vi "SSS_TX_GENERATE (SubVI).vi"(4 "초기 위상":dbl format="%#_13g", 6 "Start Frequency(Hz)":dbl=430000.0 format="%#_6p", 7 "Bandwidth":dbl=40000.0 format="%#_6p", 9 "sampling rate":dbl=3760000.0 caption="Sampling Frequency" format="%0.2f", 10 "Pulse length(sec)":dbl=4e-06, 11 "STEP":i32=100) -> (1 "TX.CH1 2":waveform(dbl)(graph), 2 "TX Spectrum":cluster{"f0":dbl, "df":dbl, "magnitude":dbl[]}(graph), 3 "TX.CH1":waveform(dbl)(graph), 5 "Hz/1STEP":dbl)   [LabVIEW 2017]
uses:
  <vilib>/measure/maspectr.llb/FFT Power Spectrum and PSD for 1 Chan.vi
  <vilib>/Analysis/NI_AALBase.lvlib
  <vilib>/measure/NI_MAPro.lvlib
panel:
  out "크기 2":i32
  out "크기":i32
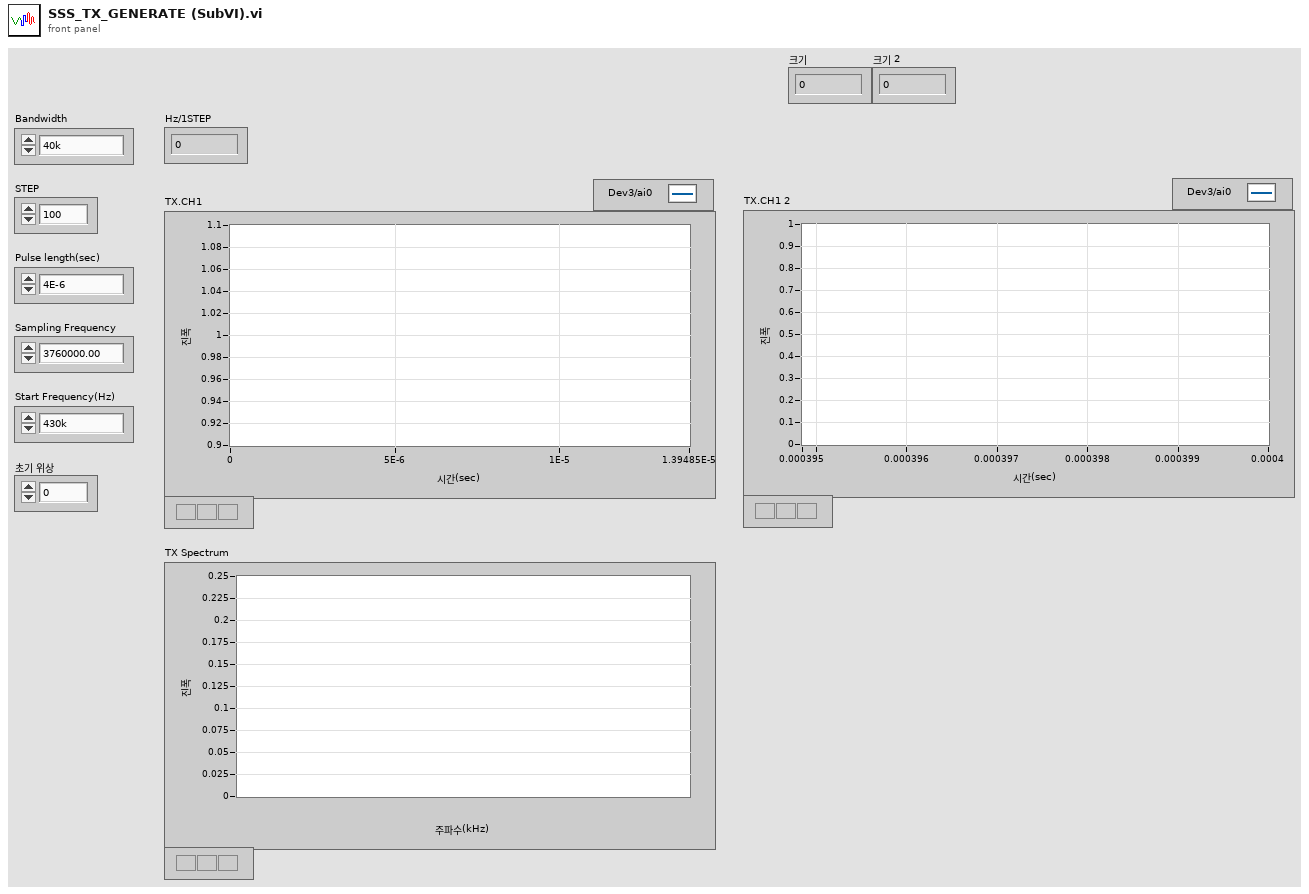
[diagram p1: front panel]
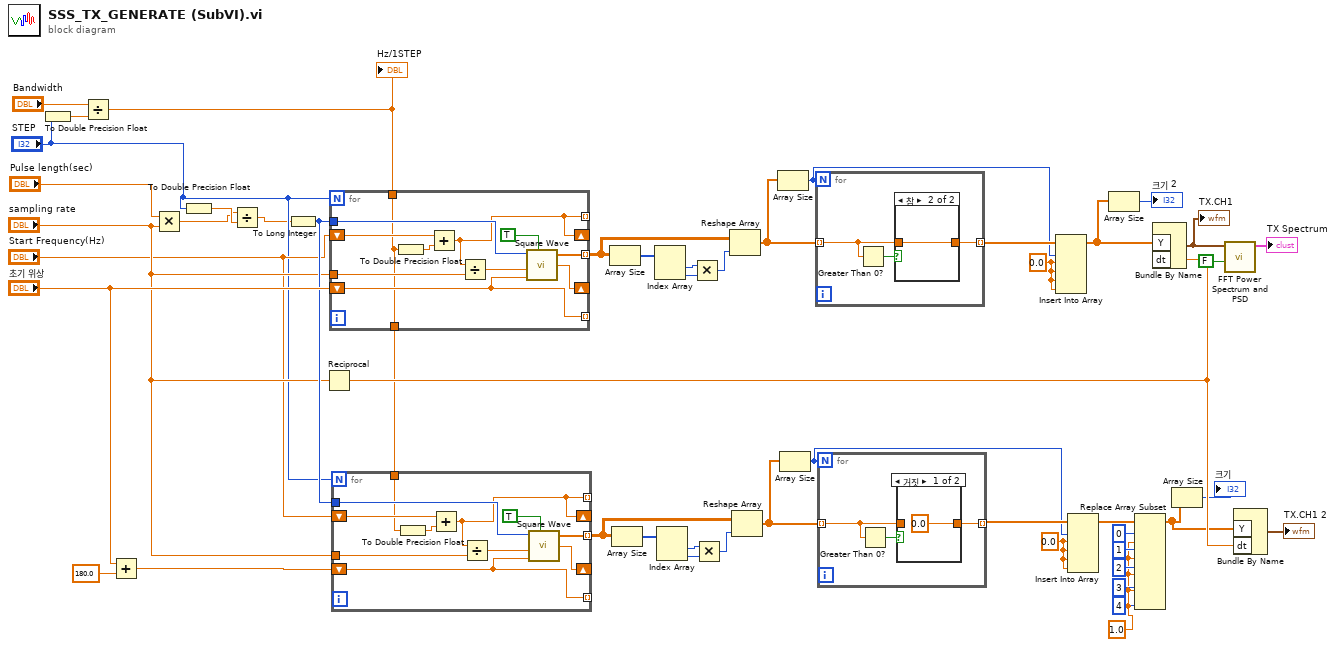
[diagram p0: block diagram]
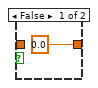
[diagram p3: hidden frame]
diagram:
  w9 = 1.0 ("새 원소/부분배열")
  w18 = 0.0 ("새 원소/부분배열")
  w19 = 0.0 ("새 원소/부분배열")
  n1 = To Double Precision Float(number="STEP") -> (double precision float=w33:dbl)
  n2 = Divide(x="Bandwidth", y=w33) -> (x/y=w34:dbl)
  "Hz/1STEP" <- w34
  n3 = Add(x="초기 위상", y=180.0) -> (x+y=w47:dbl)
  n4 = Multiply(x="Pulse length(sec)", y="sampling rate") -> (x*y=w2:dbl)
  n5 = To Double Precision Float(number="STEP") -> (double precision float=w3:dbl)
  n6 = Divide(x=w2, y=w3) -> (x/y=w1:dbl)
  n7 = To Long Integer(number=w1) -> (32bit integer=w43:i32)
  n8 = Reciprocal(x="sampling rate") -> (1/x=w48:dbl)
  n9 = for {
    N: "STEP" -> [_]
    tunnel: w43 -> [w60]
    shift-right: [w58] -> _
    shift-left: "초기 위상" -> [w51]
    tunnel: [w57] -> w25 mode=indexing
    shift-right: [w52] -> _
    shift-left: "Start Frequency(Hz)" -> [w56]
    tunnel: "sampling rate" -> [w54]
    tunnel: [w52] -> _ mode=indexing
    tunnel: [w51] -> _ mode=indexing
    tunnel: w34 -> [w50]
    tunnel: [w50] -> w44
    n10 = To Double Precision Float(number=w50) -> (double precision float=w55:dbl)
    n11 = Add(x=w56, y=w55) -> (x+y=w52:dbl)
    n12 = Divide(x=w52, y=w54) -> (x/y=w53:dbl)
    n13 = call <vilib>:"Square Wave.vi"("samples"=w60, "reset phase"=TRUE, "frequency"=w53, "phase in"=w51) -> ("square wave"=w57:dbl[], "phase out"=w58:dbl)  [unwired: 2 in, 1 out]
  }
  n14 = for {
    N: "STEP" -> [_]
    tunnel: w43 -> [w71]
    shift-right: [w69] -> _
    shift-left: w47 -> [w62]
    tunnel: [w68] -> w37 mode=indexing
    shift-right: [w63] -> _
    shift-left: "Start Frequency(Hz)" -> [w67]
    tunnel: "sampling rate" -> [w65]
    tunnel: [w63] -> _ mode=indexing
    tunnel: [w62] -> _ mode=indexing
    tunnel: w44 -> [w61]
    n15 = To Double Precision Float(number=w61) -> (double precision float=w66:dbl)
    n16 = Add(x=w67, y=w66) -> (x+y=w63:dbl)
    n17 = Divide(x=w63, y=w65) -> (x/y=w64:dbl)
    n18 = call <vilib>:"Square Wave.vi"("samples"=w71, "reset phase"=TRUE, "frequency"=w64, "phase in"=w62) -> ("square wave"=w68:dbl[], "phase out"=w69:dbl)  [unwired: 2 in, 1 out]
  }
  n19 = Array Size(array=w25) -> (size(s)=w24:i32[])
  n20 = Array Size(array=w37) -> (size(s)=w36:i32[])
  n21 = Index Array(array=w24) -> (element #1=w26:i32, element #2=w27:i32)  [unwired: 2 in]
  n22 = Index Array(array=w36) -> (element #1=w38:i32, element #2=w39:i32)  [unwired: 2 in]
  n23 = Multiply(x=w26, y=w27) -> (x*y=w23:i32)
  n24 = Multiply(x=w38, y=w39) -> (x*y=w35:i32)
  n25 = Reshape Array(w25, w23) -> (w31:dbl[])
  n26 = Reshape Array(w37, w35) -> (w40:dbl[])
  n27 = Array Size(array=w31) -> (size(s)=w20:i32)
  n28 = Array Size(array=w40) -> (size(s)=w16:i32)
  n29 = for {
    N: w20 -> [_]
    tunnel: w31 -> [w73] mode=indexing
    tunnel: [w72] -> w21 mode=indexing
    n30 = Greater Than 0?(x=w73) -> (x > 0?=w74:bool)
    n31 = case shown="참" w74 {
      tunnel: w73 -> [_ w76]
      tunnel: [0.0 w76] -> w72
      frame False {
      }
      frame True {
      }
    }
  }
  n32 = for {
    N: w16 -> [_]
    tunnel: w40 -> [w78] mode=indexing
    tunnel: [w77] -> w17 mode=indexing
    n33 = Greater Than 0?(x=w78) -> (x > 0?=w79:bool)
    n34 = case shown="거짓" w79 {
      tunnel: w78 -> [_ w81]
      tunnel: [0.0 w81] -> w77
      frame False {
      }
      frame True {
      }
    }
  }
  n35 = Insert Into Array(array=w21, index=w20, new element #1=w19, new element #2=w19, new element #3=w19, new element #4=w19) -> (w6:dbl[])
  n36 = Insert Into Array(array=w17, index=w16, new element #1=w18, new element #2=w18, new element #3=w18, new element #4=w18) -> (w15:dbl[])
  n37 = Array Size(array=w6) -> (size(s)=→"크기 2":i32)
  n38 = Replace Array Subset(array=w15, new element #1=w9, index #1=0 ("인덱스"), new element #2=w9, index #2=1 ("인덱스"), new element #3=w9, index #3=2 ("인덱스"), new element #4=w9, index #4=3 ("인덱스"), new element #5=w9, index #5=4 ("인덱스")) -> (w8:dbl[])
  n39 = Bundle By Name("Y"=w6, "dt"=w48) -> (w29:waveform(dbl))  [unwired: 1 in]
  "TX.CH1" <- w29
  n40 = Array Size(array=w8) -> (size(s)=→"크기":i32)
  n41 = call-poly <vilib>:"FFT Power Spectrum and PSD.vi"("dB On (F)"=FALSE, "time signal"=w29) -> ("Power Spectrum / PSD"=→"TX Spectrum":cluster{"f0":dbl, "df":dbl, "magnitude":dbl[]})  [unwired: 6 in, 3 out]
  n42 = Bundle By Name("Y"=w8, "dt"=w48) -> (→"TX.CH1 2":waveform(dbl))  [unwired: 1 in]
